vi "MEASURE_2dmapping-2.vi"() -> ()   [LabVIEW 2021]
uses:
  <vilib>/Math Plots/3D Math Plots/3D Surface/3D Surface XCtrl/3D Surface.xctl
  <vilib>/Math Plots/3D Math Plots/3D Surface/3D Surface Datatype/3D Surface Datatype.lvclass
  <instrlib>/Keithley 24XX/Public/Data/Read (Multiple Points).vi
  <vilib>/Utility/file.llb/Write To Spreadsheet File (DBL).vi
  <vilib>/Math Plots/3D Math Plots/3D Surface/3D Surface Datatype/Public/Plot Helper (Vector).vi
  <instrlib>/Stanford Research 830/Stanford Research 830.lvlib
  <instrlib>/Keithley 2450/Keithley 2450.lvlib
  <instrlib>/Keithley 24XX/Keithley 24XX.lvlib
  <vilib>/Analysis/NI_AALBase.lvlib
panel:
  in  "manual phase 2":dbl=1.0
  in  "auto phase 2":bool=TRUE
  in  "harmonic 2":dbl=1.0
  in  "Sine Output Amplitude (1 V) 3":dbl=0.05
  in  "Input Connection (0: Single-Ended Voltage)  2":u16(ring) items=["Single-Ended Voltage", "Differential Voltage", "1 MOhm Current Gain", "100 MOhm Current Gain"]
  in  "frequency 2":dbl=50.0 format="%#_13g"
  in  "manual phase":dbl=1.0
  in  "auto phase":bool=TRUE
  in  "harmonic":dbl=1.0
  in  "LOCKIN address 2":refnum<visa-resource-name>="GPIB0::8::INSTR"
  in  "GATE / SD stablization 5":dbl=0.1 format="%#_13g"
  in  "GATE / SD stablization 4":dbl=0.1 format="%#_13g"
  in  "ramping step":i32=20
  in  "Compliance  Level (1uA) 2":dbl=1e-08
  in  "Source Mode  (0: Voltage) 2":u16(ring) items=["Voltage", "Current"]
  out "3D Surface":refnum<class "3D Plot Datatype.lvclass">[](xcontrol)
  in  "scaning step2":i32=60
  out "gate voltage1":dbl=3.0 format="%#_13g"
  in  "scanning step1":i32=30
  in  "GATE2 end Value   2":dbl=10.0
  in  "GATE2 starting Value  2":dbl=-14.0
  out "gate 2leaking":dbl=1.1399661770106206e-10
  out "gate voltage2":dbl=10.0 format="%#_13g"
  in  "Serial Configuration":T1={"Baud Rate"=9600, "Parity"=0, "Data Bits"=8, "Stop Bits"=10, "Flow Control"=0} {"Flow Control" items=["None", "XON/XOFF", "RTS/CTS", "XON/XOFF & RTS/CTS", "DTR/DSR", "XON/XOFF & DTR/DSR"]; "Stop Bits" items=["1.0"=10, "1.5"=15, "2.0"=20]; "Data Bits" items=["7"=7, "8"=8]; "Parity" items=["None", "Odd", "Even", "Mark", "Space"]; "Baud Rate" items=["300"=300, "600"=600, "1200"=1200, "2400"=2400, "4800"=4800, "9600"=9600, "19200"=19200]}
  in  "gate2 address":refnum<visa-resource-name>="GPIB0::25::INSTR"
  in  "Save data or not":bool=TRUE
  in  "path (folder + filename)":string="C:\\Users\\User\\Data\\Jason\\03282019\\mapping_3"
  out "XY Graph":cluster{dbl[], dbl[]}(graph)={[-14.0, -13.6, -13.2, -12.8, -12.4, -12.0, -11.6, -11.2, -10.8, -10.4, -10.0, -9.6, -9.2, -8.8, -8.399999999999999, -8.0, -7.6, -7.199999999999999, -6.8, -6.3999999999999995, -6.0, -5.6, -5.199999999999999, -4.799999999999999, -4.399999999999999, -4.0, -3.5999999999999996, -3.1999999999999993, -2.799999999999999, -2.3999999999999986, -2.0, -1.5999999999999996, -1.1999999999999993, -0.7999999999999989, -0.3999999999999986, 0.0, 0.40000000000000036, 0.8000000000000007, 1.200000000000001, 1.6000000000000014, 2.0, 2.400000000000002, 2.8000000000000007, 3.1999999999999993, 3.6000000000000014, 4.0, 4.400000000000002, 4.800000000000001, 5.200000000000003, 5.600000000000001, 6.0, 6.400000000000002, 6.800000000000001, 7.200000000000003, 7.600000000000001, 8.0, 8.400000000000002, 8.8, 9.200000000000003, 9.600000000000001, 10.0], [0.000948314, 0.000947837, 0.000947598, 0.000947479, 0.000947241, 0.000946883, 0.000946645, 0.000945572, 0.000944141, 0.000942711, 0.000941519, 0.000939969, 0.000938658, 0.000937108, 0.00093532, 0.000933651, 0.000931863, 0.000929955, 0.000928048, 0.000926021, 0.000923995, 0.00092173, 0.000919465, 0.0009172, 0.000914697, 0.000912312, 0.000909809, 0.000907306, 0.000904683, 0.00090218, 0.000899557, 0.000896934, 0.000894193, 0.00089157, 0.000888947, 0.000886325, 0.000883702, 0.00088108, 0.000878457, 0.000875834, 0.000873331, 0.000870828, 0.000868324, 0.00086594, 0.000863437, 0.000861172, 0.000858787, 0.000856522, 0.000854257, 0.000852112, 0.000849966, 0.000847939, 0.000846032, 0.000844125, 0.000842217, 0.000840429, 0.000838879, 0.000837211, 0.000835661, 0.00083435, 0.000833277]}
  out "LOCKIN Measurement":dbl=0.000833277
  in  "Parameter (1: X)":u16(ring)=1 items=["X"=1, "Y"=2, "R"=3, "Theta"=4, "Channel 1"=5, "Channel 2"=6, "Aux In 1"=7, "Aux In 2"=8, "Aux In 3"=9, "Aux In 4"=10]
  out "gate leaking":string="4.458176E-12\n"
  in  "GATE1 end Value (default 0)":dbl=3.0
  in  "GATE1 starting(small) Value":dbl=-3.0
  in  "Function (0: Volts) 2":u16(ring) items=["Volts", "Current", "Resistance"]
  in  "Source Compaliance":dbl=1e-08
  in  "gate1 address":refnum<visa-resource-name>="GPIB0::18::INSTR"
  in  "SD stabilization(S) 2":dbl=0.1 format="%#_13g"
  in  "Sine Output Amplitude (1 V) 2":dbl=0.05
  in  "GATE / SD stablization 3":dbl=0.2 format="%#_13g"
  in  "frequency":dbl=50.0 format="%#_13g"
  in  "Input Connection (0: Single-Ended Voltage)":u16(ring) items=["Single-Ended Voltage", "Differential Voltage", "1 MOhm Current Gain", "100 MOhm Current Gain"]
  in  "LOCKIN address":refnum<visa-resource-name>="GPIB0::8::INSTR"
  # "Lock-in"
  # "2450 Gate Setting"
  # "2401 Gate Setting"
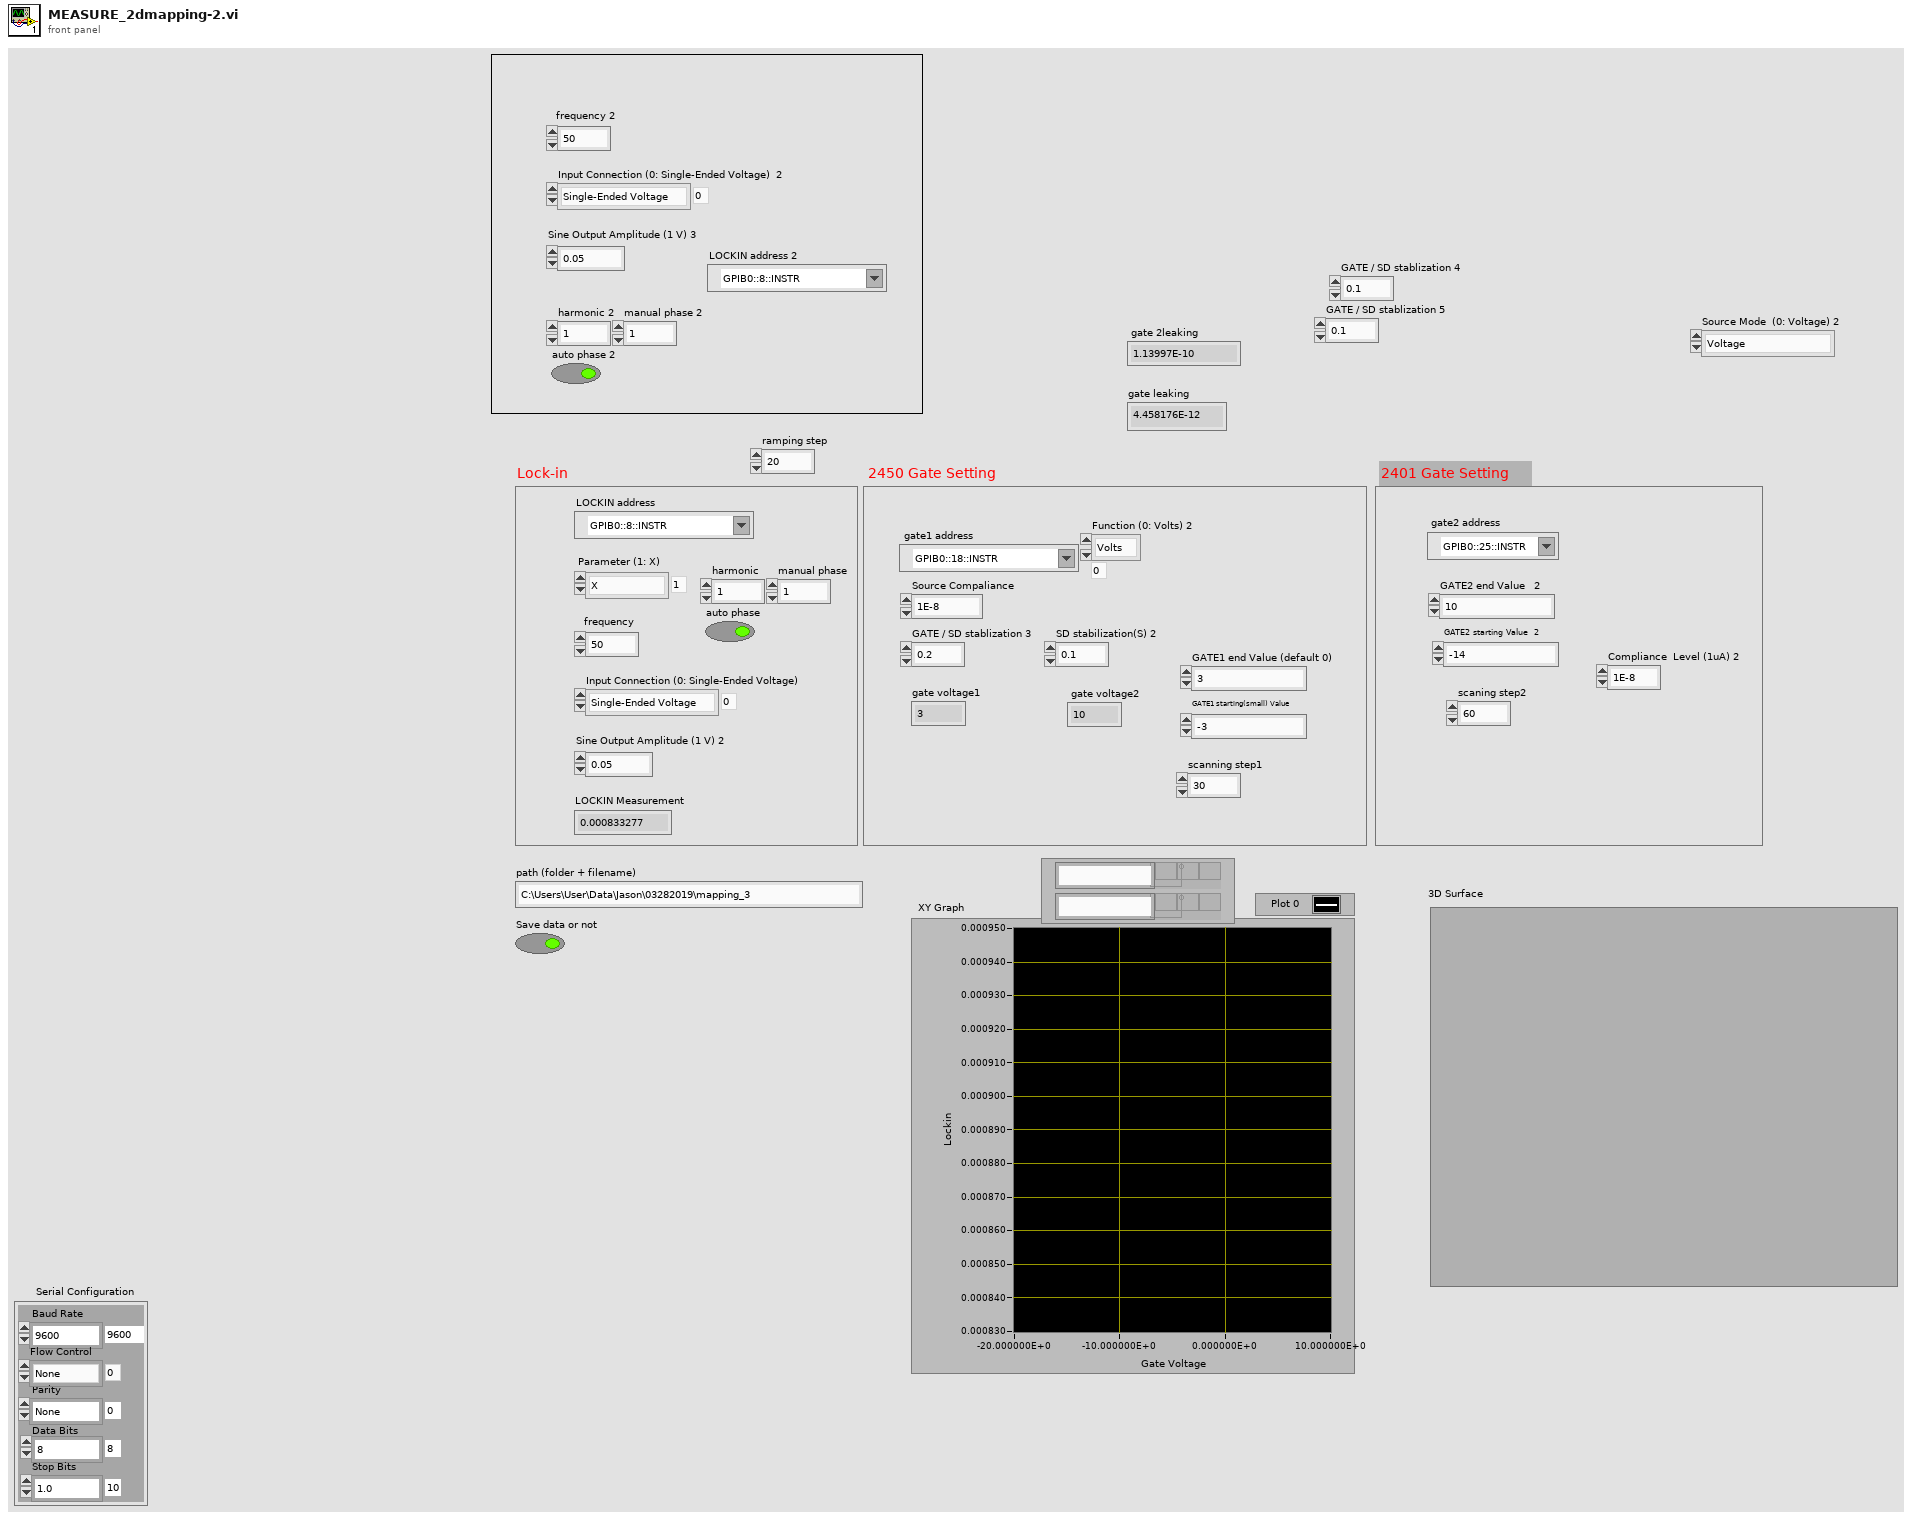
[diagram p1: front panel]
types:
  T1 = cluster{"Baud Rate":u32, "Parity":u16, "Data Bits":u16, "Stop Bits":u16, "Flow Control":u16}
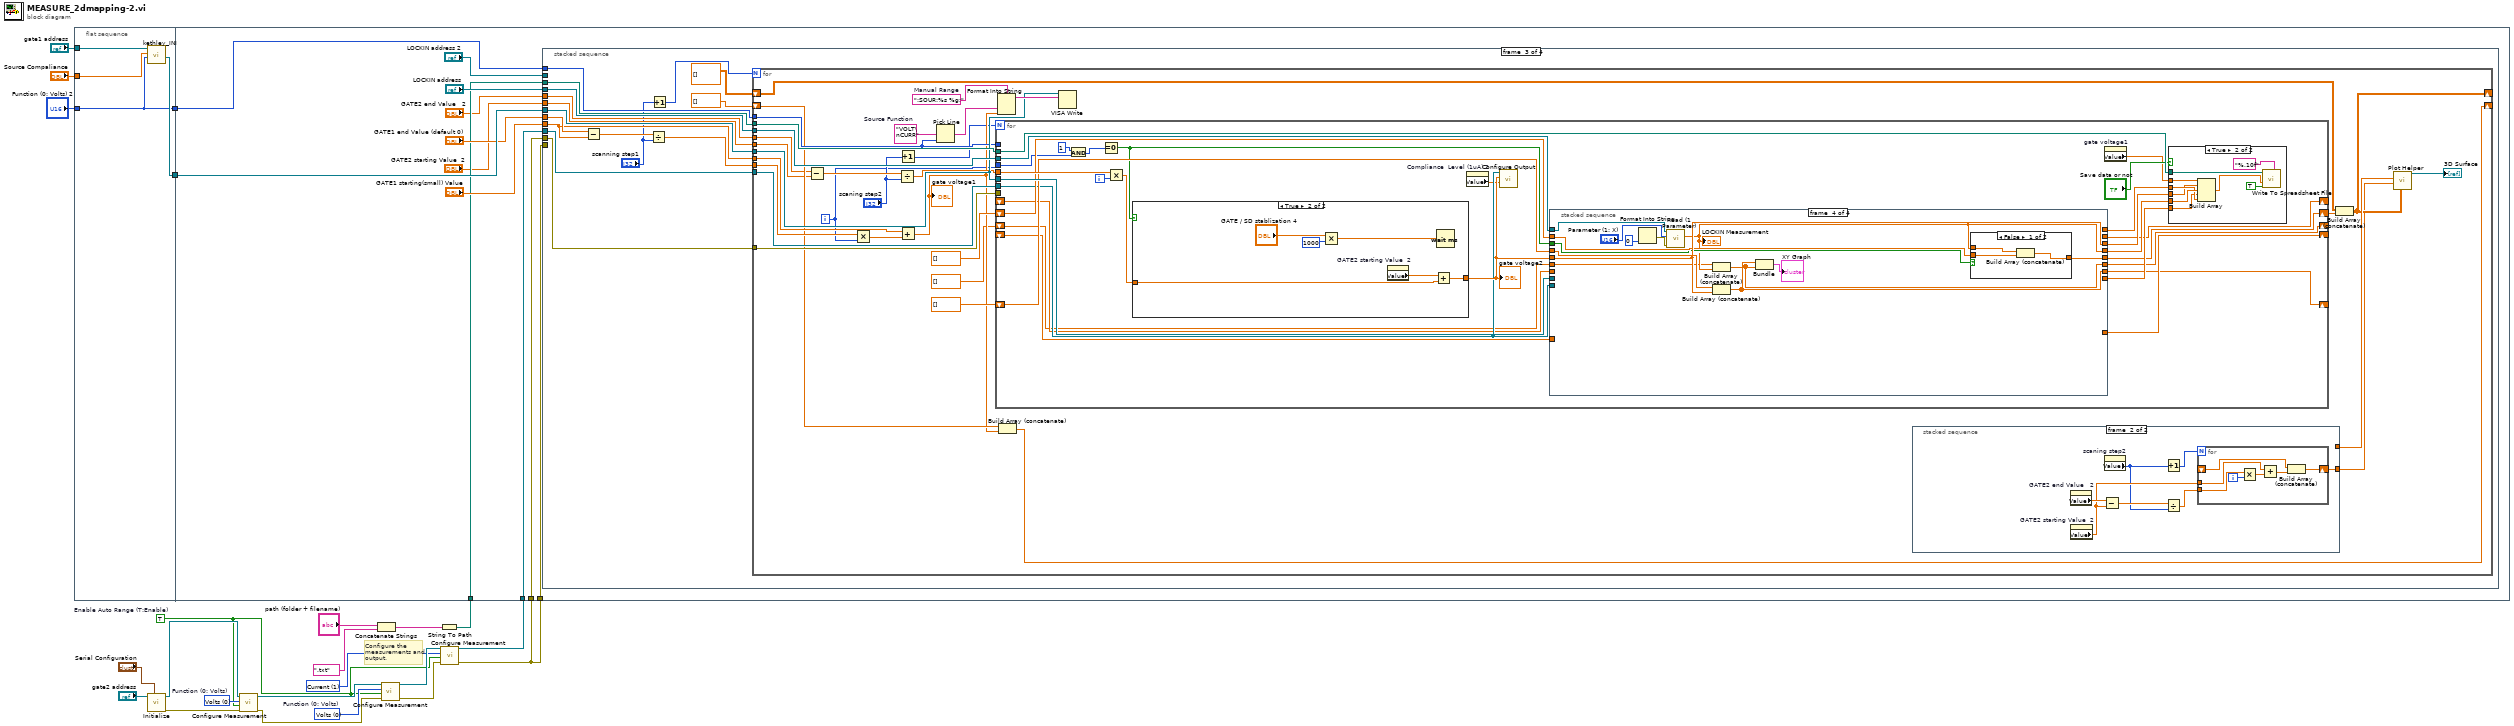
[diagram p0: block diagram]
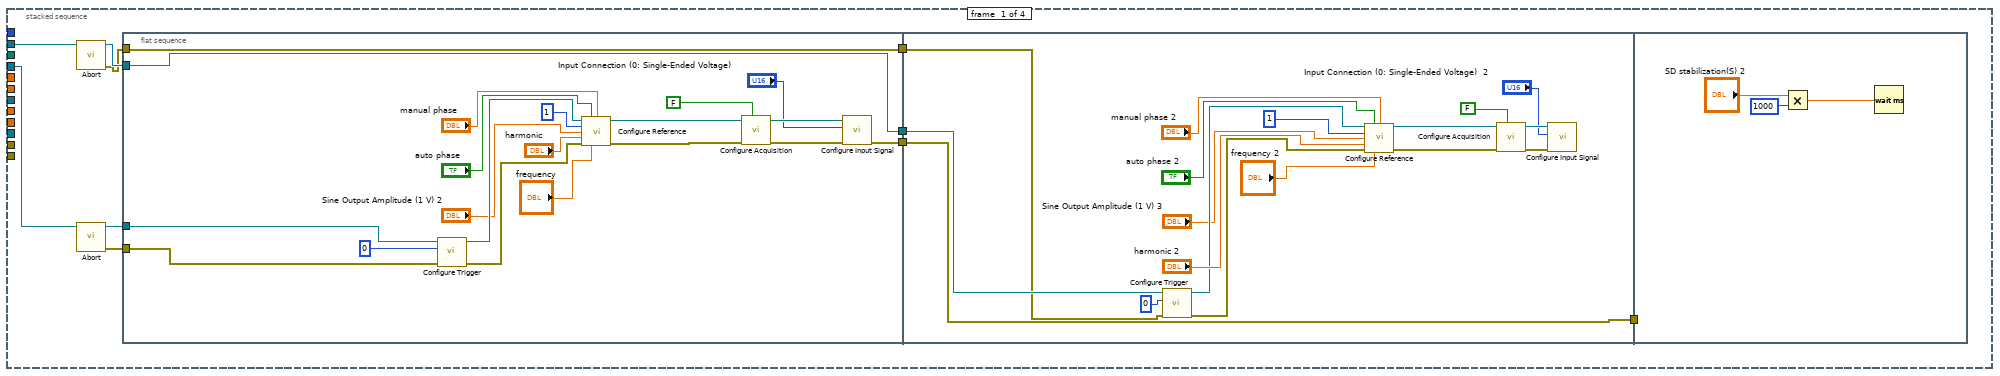
[diagram p2: hidden frame]
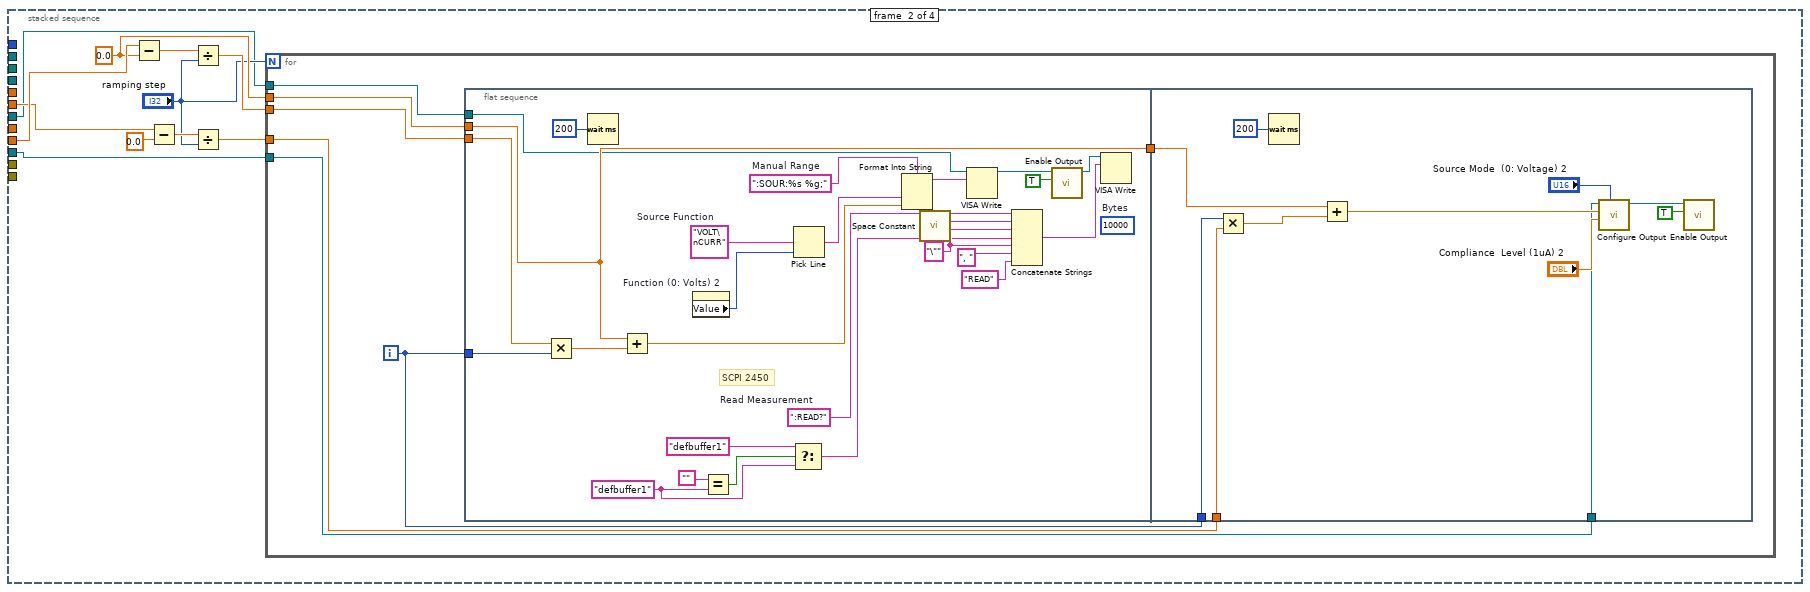
[diagram p3: hidden frame]
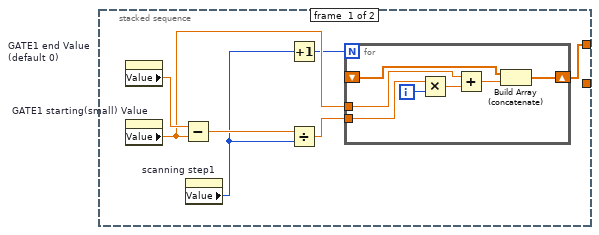
[diagram p4: hidden frame]
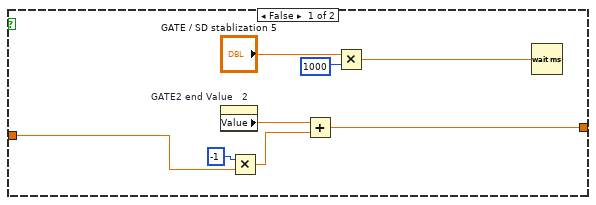
[diagram p5: hidden frame]
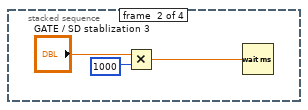
[diagram p8: hidden frame]
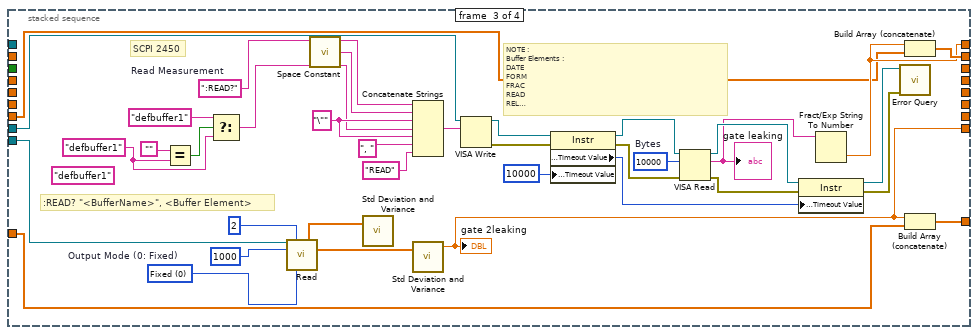
[diagram p9: hidden frame]
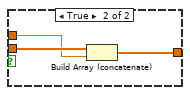
[diagram p10: hidden frame]
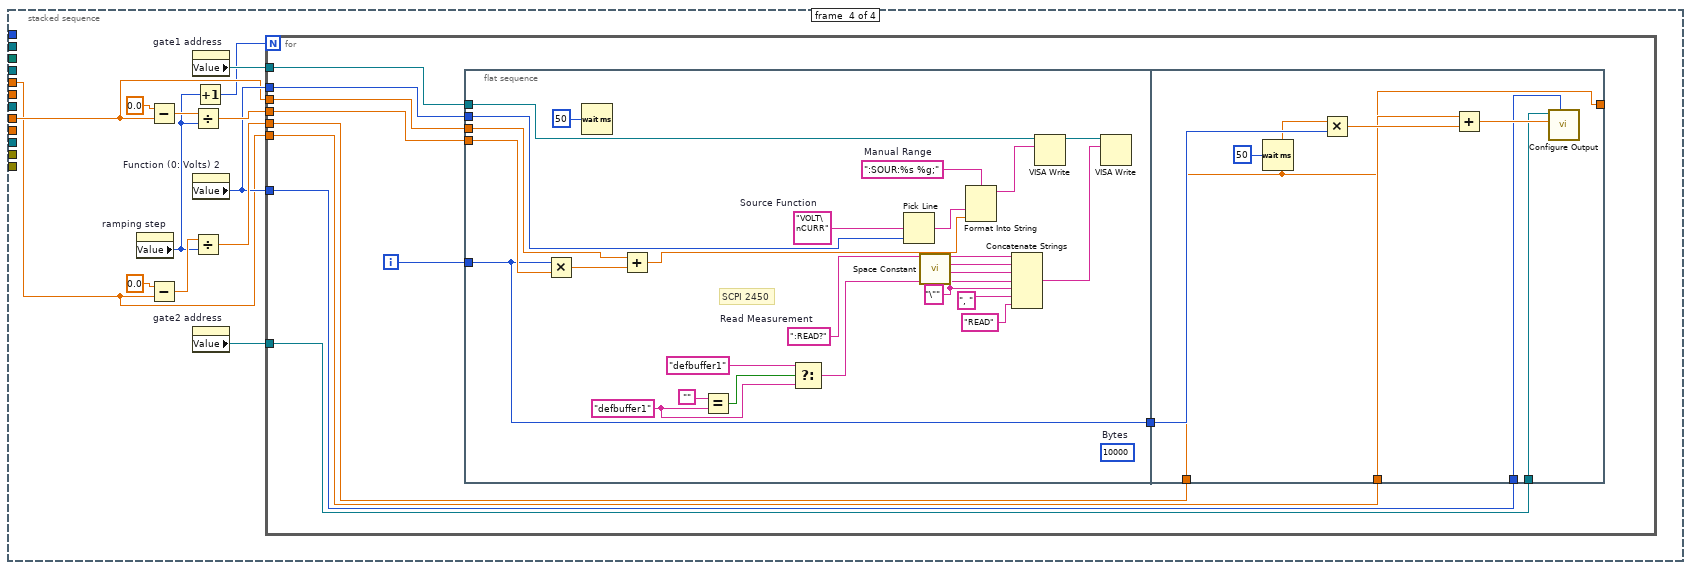
[diagram p11: hidden frame]
diagram:
  w3 = u16 1 items=["Volts", "Current", "Resistance"] ("Function (0: Volts)")
  w4 = TRUE  # Enable Auto Range (T:Enable)
  w7 = u16 0 items=["Volts", "Current", "Resistance"]  # Function (0: Volts)
  w8 = u16 0 items=["Volts", "Current", "Resistance"]  # Function (0: Volts)
  # "Configure the measurements and output."
  n1 = flat-sequence {
    tunnel: "gate1 address" -> [w27]
    tunnel: "Source Compaliance" -> [w26]
    tunnel: "Function (0: Volts) 2" -> [w24]
    tunnel: [w25] -> w20
    tunnel: [w24] -> w19
    tunnel: w20 -> [w38]
    tunnel: w19 -> [w37]
    tunnel: w15 -> [w34]
    tunnel: w2 -> [w33]
    tunnel: w1 -> [w32]
    tunnel: w1 -> [w29]
    frame #0 {
      n2 = call "kethley_INI.vi"("Function (0: Volts) in"=w24, "Source Compaliance"=w26, "VISA Refnum in"=w27) -> ("VISA resource name out"=w25:refnum<visa-resource-name>)  [unwired: 8 in]
    }
    frame #1 {
      n3 = stacked-sequence {
        tunnel: "LOCKIN address" -> [w49 _ w161 _]
        tunnel: w38 -> [_ w92 w158 _]
        tunnel: w37 -> [_ _ w157 _]
        tunnel: "GATE1 starting(small) Value" -> [_ w99 w151 _]
        tunnel: "GATE1 end Value (default 0)" -> [_ _ w152 w337]
        tunnel: w34 -> [_ _ w160 _]
        tunnel: w33 -> [_ w91 w156 _]
        tunnel: w32 -> [_ _ w159 _]
        tunnel: "GATE2 starting Value  2" -> [_ w94 w149 _]
        tunnel: "GATE2 end Value   2" -> [_ _ w150 w335]
        tunnel: w29 -> [_ _ _ _]
        tunnel: "LOCKIN address 2" -> [w43 _ _ _]
        frame #0 {
          n4 = call <instrlib>:"Abort.vi"("VISA resource name"=w43) -> ("error out"=w40:errorcluster, "VISA resource name out"=w42:refnum<visa-resource-name>)  [unwired: 9 in]
          n5 = call <instrlib>:"Abort.vi"("VISA resource name"=w49) -> ("error out"=w47:errorcluster, "VISA resource name out"=w48:refnum<visa-resource-name>)  [unwired: 9 in]
          n6 = flat-sequence {
            tunnel: w48 -> [w69]
            tunnel: [w54] -> w46
            tunnel: w47 -> [w53]
            tunnel: w42 -> [w51]
            tunnel: [w51] -> w44
            tunnel: [w50] -> w41
            tunnel: w40 -> [w50]
            tunnel: w46 -> [w87]
            tunnel: [w87] -> w45
            tunnel: w44 -> [w71]
            tunnel: w41 -> [w70]
            tunnel: w45 -> [_]
            frame #0 {
              n7 = call <instrlib>:"Configure Trigger.vi"("error in (no error)"=w53, "Trigger Source (0: Internal)"=0, "VISA resource name"=w69) -> ("error out"=w63:errorcluster, "VISA resource name out"=w64:refnum<visa-resource-name>)  [unwired: 7 in]
              n8 = call <instrlib>:"Configure Reference.vi"("VISA resource name"=w64, "Auto Phase (T: Enabled)"="auto phase", "Manual Phase (0 Degree)"="manual phase", "Reference Source (1: Internal)"=1, "Sine Output Amplitude (1 V)"="Sine Output Amplitude (1 V) 2", "Detection Harmonic Number (1)"="harmonic", "error in (no error)"=w63, "Internal Reference Frequency (1000 Hz)"="frequency") -> ("VISA resource name out"=w61:refnum<visa-resource-name>, "error out"=w56:errorcluster)  [unwired: 6 in]
              n9 = call <instrlib>:"Configure Acquisition.vi"("Continuous Storage (T: Enable)"=FALSE, "error in (no error)"=w56, "VISA resource name"=w61) -> ("error out"=w55:errorcluster, "VISA resource name out"=w59:refnum<visa-resource-name>)  [unwired: 7 in]
              n10 = call <instrlib>:"Configure Input Signal.vi"("error in (no error)"=w55, "Input Connection (0: Single-Ended Voltage)"="Input Connection (0: Single-Ended Voltage)", "VISA resource name"=w59) -> ("error out"=w54:errorcluster)  [unwired: 7 in, 1 out]
            }
            frame #1 {
              n11 = call <instrlib>:"Configure Trigger.vi"("error in (no error)"=w70, "Trigger Source (0: Internal)"=0, "VISA resource name"=w71) -> ("error out"=w81:errorcluster, "VISA resource name out"=w82:refnum<visa-resource-name>)  [unwired: 7 in]
              n12 = call <instrlib>:"Configure Reference.vi"("VISA resource name"=w82, "Auto Phase (T: Enabled)"="auto phase 2", "Manual Phase (0 Degree)"="manual phase 2", "Reference Source (1: Internal)"=1, "Sine Output Amplitude (1 V)"="Sine Output Amplitude (1 V) 3", "Detection Harmonic Number (1)"="harmonic 2", "error in (no error)"=w81, "Internal Reference Frequency (1000 Hz)"="frequency 2") -> ("VISA resource name out"=w79:refnum<visa-resource-name>, "error out"=w74:errorcluster)  [unwired: 6 in]
              n13 = call <instrlib>:"Configure Acquisition.vi"("Continuous Storage (T: Enable)"=FALSE, "error in (no error)"=w74, "VISA resource name"=w79) -> ("error out"=w73:errorcluster, "VISA resource name out"=w77:refnum<visa-resource-name>)  [unwired: 7 in]
              n14 = call <instrlib>:"Configure Input Signal.vi"("error in (no error)"=w73, "Input Connection (0: Single-Ended Voltage)"="Input Connection (0: Single-Ended Voltage)  2", "VISA resource name"=w77) -> ()  [unwired: 7 in, 2 out]
            }
            frame #2 {
              n15 = Multiply(x="SD stabilization(S) 2", y=1000) -> (x*y=w90:dbl)
              n16 = Wait (ms)(milliseconds to wait=w90) -> ()  [unwired: 1 out]
            }
          }
        }
        frame #1 {
          w98 = 0.0
          n17 = Subtract(x=w99, y=w98) -> (x-y=w101:dbl)
          n18 = Subtract(x=w94, y=0.0) -> (x-y=w97:dbl)
          n19 = Divide(x=w101, y="ramping step") -> (x/y=w100:dbl)
          n20 = Divide(x=w97, y="ramping step") -> (x/y=w93:dbl)
          n21 = for {
            N: "ramping step" -> [_]
            tunnel: w100 -> [w108]
            tunnel: w98 -> [w107]
            tunnel: w93 -> [w106]
            tunnel: w92 -> [w103]
            tunnel: w91 -> [w102]
            i -> [w105]
            n22 = flat-sequence {
              tunnel: w105 -> [w128]
              tunnel: w108 -> [w127]
              tunnel: w107 -> [w126]
              tunnel: [w126] -> w104
              tunnel: w103 -> [w124]
              tunnel: w106 -> [w142]
              tunnel: w105 -> [w141]
              tunnel: w104 -> [w140]
              tunnel: w102 -> [w138]
              frame #0 {
                w109 = "defbuffer1" ("Buffer Name (defbuffer1) 2")
                w117 = "\""
                w114 = ":READ?"  # Read Measurement
                (unwired) u32 10000  # Bytes
                w133 = "VOLT\nCURR"  # Source Function
                w132 = ":SOUR:%s %g;"  # Manual Range
                # "SCPI 2450"
                n23 = Multiply(x=w127, y=w128) -> (x*y=w130:dbl)
                n24 = Wait (ms)(milliseconds to wait=200) -> ()  [unwired: 1 out]
                n25 = Add(x=w126, y=w130) -> (x+y=w129:dbl)
                n26 = property on="Function (0: Volts) 2" class="Ring (strict)"() -> ("Value"=w125:u16)  [unwired: 2 in, 2 out]
                n27 = Equal?(x="", y=w109) -> (x = y?=w110:bool)
                n28 = Select(t="defbuffer1", s=w110, f=w109) -> (s? t:f=w116:string)
                n29 = Pick Line(multi-line string=w133, line index=w125) -> (output string=w134:string)  [unwired: 1 out]
                n30 = Format Into String(format string=w132, w134, w129) -> (resulting string=w131:string)  [unwired: 2 in, 1 out]
                n31 = call <vilib>:"Space Constant.vi"() -> ("String"=w115:string)
                n32 = VISA Write(VISA resource name=w124, write buffer=w131) -> (VISA resource name out=w122:refnum<visa-resource-name>)  [unwired: 1 in, 2 out]
                n33 = Concatenate Strings(w114, w115, w117, w116, w117, ", " ("string"), "READ" ("Buffer Elements 2")) -> (w120:string)
                n34 = call <instrlib>:"Enable Output.vi"("Enable Output (T: Enable)"=TRUE, "VISA resource name"=w122) -> ("VISA resource name out"=w111:refnum<visa-resource-name>)  [unwired: 8 in, 1 out]
                n35 = VISA Write(VISA resource name=w111, write buffer=w120) -> ()  [unwired: 1 in, 3 out]
              }
              frame #1 {
                n36 = Multiply(x=w141, y=w142) -> (x*y=w143:dbl)
                n37 = Wait (ms)(milliseconds to wait=200) -> ()  [unwired: 1 out]
                n38 = Add(x=w140, y=w143) -> (x+y=w144:dbl)
                n39 = call <instrlib>:"Configure Output.vi"("Source Mode  (0: Voltage)"="Source Mode  (0: Voltage) 2", "Compliance  Level (0.1)"="Compliance  Level (1uA) 2", "Output Level (0)"=w144, "VISA resource name"=w138) -> ("VISA resource name out"=w135:refnum<visa-resource-name>)  [unwired: 6 in, 1 out]
                n40 = call <instrlib>:"Enable Output.vi"("Enable Output (T: Enable)"=TRUE, "VISA resource name"=w135) -> ()  [unwired: 8 in, 2 out]
              }
            }
          }
        }
        frame #2 {
          n41 = Subtract(x=w152, y=w151) -> (x-y=w155:dbl)
          n42 = Divide(x=w155, y="scanning step1") -> (x/y=w154:dbl)
          n43 = Increment(x="scanning step1") -> (x+1=w147:i32)
          n44 = for {
            N: w147 -> [_]
            tunnel: w157 -> [w181]
            tunnel: w158 -> [w182]
            tunnel: w161 -> [w193]
            tunnel: w160 -> [w192]
            tunnel: w159 -> [w191]
            tunnel: w156 -> [w190]
            tunnel: w151 -> [w189]
            tunnel: w154 -> [w188]
            shift-right: [w164] -> _
            shift-left: dbl[] [] ("appended array") -> [w176]
            tunnel: w150 -> [w173]
            tunnel: w149 -> [w172]
            shift-right: [w165] -> _
            shift-left: dbl[][] [] ("Intensity Graph") -> [w166]
            i -> [w169]
            w184 = "VOLT\nCURR"  # Source Function
            w185 = ":SOUR:%s %g;"  # Manual Range
            n45 = Subtract(x=w173, y=w172) -> (x-y=w180:dbl)
            n46 = Multiply(x=w188, y=w169) -> (x*y=w187:dbl)
            n47 = Divide(x=w180, y="scaning step2") -> (x/y=w179:dbl)
            n48 = Increment(x="scaning step2") -> (x+1=w170:i32)
            n49 = Add(x=w189, y=w187) -> (x+y=w175:dbl)
            "gate voltage1" <- w175
            n50 = Pick Line(multi-line string=w184, line index=w181) -> (output string=w183:string)  [unwired: 1 out]
            n51 = for {
              N: w170 -> [_]
              tunnel: w181 -> [_]
              tunnel: w182 -> [w250]
              tunnel: w193 -> [w249]
              tunnel: w192 -> [w246]
              tunnel: w191 -> [_]
              tunnel: w190 -> [w234]
              shift-right: [w237] -> _
              shift-left: _ -> [w224]
              tunnel: w179 -> [w243]
              shift-right: [w239] -> w174
              shift-left: dbl[] [] ("appended array") -> [w240]
              shift-right: [w227] -> _
              shift-left: dbl[] [] ("appended array") -> [w238]
              shift-right: [w233] -> _
              shift-left: _ -> [w232]
              tunnel: w169 -> [w228]
              shift-right: [w225] -> _
              shift-left: dbl[] [] ("appended array") -> [w223]
              i -> [w230]
              n52 = And(x=1, y=w228) -> (x .and. y?=w229:i32)
              n53 = Equal To 0?(x=w229) -> (x = 0?=w226:bool)
              n54 = Multiply(x=w243, y=w230) -> (x*y=w242:dbl)
              n55 = case shown="True" w226 {
                tunnel: w242 -> [w258 w259]
                tunnel: [w254 w263] -> w241
                frame False {
                  n56 = property on="GATE2 end Value   2" class="DigNum (strict)"() -> ("Value"=w255:dbl)  [unwired: 2 in, 2 out]
                  n57 = Multiply(x=-1, y=w258) -> (x*y=w256:dbl)
                  n58 = Add(x=w255, y=w256) -> (x+y=w254:dbl)
                  n59 = Multiply(x="GATE / SD stablization 5", y=1000) -> (x*y=w253:dbl)
                  n60 = Wait (ms)(milliseconds to wait=w253) -> ()  [unwired: 1 out]
                }
                frame True {
                  n61 = Multiply(x="GATE / SD stablization 4", y=1000) -> (x*y=w262:dbl)
                  n62 = property on="GATE2 starting Value  2" class="DigNum (strict)"() -> ("Value"=w264:dbl)  [unwired: 2 in, 2 out]
                  n63 = Add(x=w264, y=w259) -> (x+y=w263:dbl)
                  n64 = Wait (ms)(milliseconds to wait=w262) -> ()  [unwired: 1 out]
                }
              }
              "gate voltage2" <- w241
              n65 = property on="Compliance  Level (1uA) 2" class="DigNum (strict)"() -> ("Value"=w222:dbl)  [unwired: 2 in, 2 out]
              n66 = call <instrlib>:"Configure Output.vi"("Compliance  Level (0.1)"=w222, "Output Level (0)"=w241, "VISA resource name"=w234) -> ()  [unwired: 7 in, 2 out]
              n67 = stacked-sequence {
                tunnel: w250 -> [_ _ w290 _]
                tunnel: w249 -> [_ _ _ w323]
                tunnel: [_ _ w289 _] -> w233
                tunnel: w240 -> [_ _ _ w318]
                tunnel: [_ _ _ w317] -> w239
                tunnel: [_ _ _ w321] -> w227
                tunnel: [_ _ _ w315] -> w248
                tunnel: [_ _ w287 _] -> w247
                tunnel: [_ _ w281 _] -> w237
                tunnel: w224 -> [_ _ w280 _]
                tunnel: [_ _ w279 _] -> w244
                tunnel: w241 -> [_ _ _ w319]
                tunnel: w238 -> [_ _ _ w320]
                tunnel: [_ _ _ w319] -> w236
                tunnel: w234 -> [_ _ w277 _]
                tunnel: w232 -> [_ _ w278 _]
                tunnel: w226 -> [_ _ _ w316]
                tunnel: [_ _ _ w313] -> w225
                tunnel: w223 -> [_ _ _ w314]
                frame #0 {
                }
                frame #1 {
                  n68 = Multiply(x="GATE / SD stablization 3", y=1000) -> (x*y=w276:dbl)
                  n69 = Wait (ms)(milliseconds to wait=w276) -> ()  [unwired: 1 out]
                }
                frame #2 {
                  w284 = u16 0 items=["Fixed", "Sweep", "List"]  # Output Mode (0: Fixed)
                  w301 = "defbuffer1" ("Buffer Name (defbuffer1) 2")
                  (unwired) "defbuffer1" ("t")
                  w299 = "\""
                  w296 = ":READ?"  # Read Measurement
                  w305 = u32 10000  # Bytes
                  # "NOTE :\nBuffer Elements :\nDATE\nFORM\nFRAC\nREAD\nREL\nSEC\nSOUR\nSOURFORM\nSOURSTAT\nSOURUNIT\nSTAT\nTIME\nTsT\nUNIT"
                  # ":READ? \"<BufferName>\", <Buffer Element>"
                  # "SCPI 2450"
                  n70 = Equal?(x="", y=w301) -> (x = y?=w302:bool)
                  n71 = Select(t="defbuffer1", s=w302, f=w301) -> (s? t:f=w298:string)
                  n72 = call-poly <instrlib>:"Read.vi"("VISA resource name"=w277, "Sample Count (1)"=u32 2 ("Number of Samples"), "Timeout (10000 ms)"=1000, "Output Mode (0: Fixed)"=w284) -> ("Voltage"=w282:sgl[], "Current"=w283:sgl[])  [unwired: 5 in, 5 out]
                  n73 = call <vilib>:"Space Constant.vi"() -> ("String"=w297:string)
                  n74 = call <vilib>:"Std Deviation and Variance.vi"("X"=w282) -> ()  [unwired: 1 in, 3 out]
                  n75 = Concatenate Strings(w296, w297, w299, w298, w299, ", " ("string"), "READ" ("Buffer Elements 2")) -> (w312:string)
                  n76 = call <vilib>:"Std Deviation and Variance.vi"("X"=w283) -> ("mean"=w279:dbl)  [unwired: 1 in, 2 out]
                  "gate 2leaking" <- w279
                  n77 = VISA Write(VISA resource name=w290, write buffer=w312) -> (VISA resource name out=w304:refnum<visa-resource-name>, error out=w311:errorcluster)  [unwired: 1 in, 1 out]
                  n78 = property class="Instr"(reference=w304, error in=w311, "General Settings:Timeout Value"=10000 ("Timeout (10000 ms) 2")) -> (reference out=w310:refnum<visa-resource-name>, error out=w309:errorcluster, "General Settings:Timeout Value"=w306:u32)
                  n79 = VISA Read(VISA resource name=w310, byte count=w305, error in (no error)=w309) -> (VISA resource name out=w308:refnum<visa-resource-name>, read buffer=w288:string, error out=w307:errorcluster)  [unwired: 1 out]
                  "gate leaking" <- w288
                  n80 = property class="Instr"(reference=w308, error in=w307, "General Settings:Timeout Value"=w306) -> (reference out=w294:refnum<visa-resource-name>, error out=w293:errorcluster)
                  n81 = Fract/Exp String To Number(string=w288) -> (number=w287:dbl)  [unwired: 3 in, 1 out]
                  n82 = call <instrlib>:"Error Query.vi"("error in (no error)"=w293, "VISA resource name"=w294) -> ()  [unwired: 10 out]
                  n83 = Build Array (concatenate)(w287, w278) -> (w289:dbl[])
                  n84 = Build Array (concatenate)(w279, w280) -> (w281:dbl[])
                }
                frame #3 {
                  n85 = Format Into String(0) -> (error out=w326:errorcluster)  [unwired: 3 in, 1 out]
                  n86 = call <instrlib>:"Read (1 Parameter).vi"("error in (no error)"=w326, "Parameter (1: X)"="Parameter (1: X)", "VISA resource name"=w323) -> ("Measurement"=w315:dbl)  [unwired: 6 in, 2 out]
                  "LOCKIN Measurement" <- w315
                  n87 = Build Array (concatenate)(w314, w315) -> (w313:dbl[])
                  n88 = Build Array (concatenate)(w320, w319) -> (w321:dbl[])
                  n89 = Bundle(w321, w313) -> (→"XY Graph":cluster{dbl[], dbl[]})  [unwired: 1 in]
                  n90 = case shown="False" w316 {
                    tunnel: w318 -> [w328 w332]
                    tunnel: w315 -> [w329 w331]
                    tunnel: [w327 w330] -> w317
                    frame False {
                      n91 = Build Array (concatenate)(w329, w328) -> (w327:dbl[])
                    }
                    frame True {
                      n92 = Build Array (concatenate)(w332, w331) -> (w330:dbl[])
                    }
                  }
                }
              }
              n93 = property on="gate voltage1" class="DigNum (strict)"() -> ("Value"=w235:dbl)  [unwired: 2 in, 2 out]
              n94 = case shown="True" "Save data or not" {
                tunnel: w248 -> [_ w273]
                tunnel: w247 -> [_ w272]
                tunnel: w246 -> [_ w270]
                tunnel: w244 -> [_ w267]
                tunnel: w236 -> [_ w266]
                tunnel: w235 -> [_ w265]
                frame False {
                }
                frame True {
                  n95 = Build Array(w265, w266, w273, w267, w272) -> (w271:dbl[])
                  n96 = call-poly <vilib>:"Write To Spreadsheet File.vi"("format (%.3f)"="%.10f", "append to file? (new file:F)"=TRUE, "1D data"=w271, "file path (dialog if empty)"=w270) -> ()  [unwired: 4 in, 1 out]
                }
              }
            }
            n97 = Format Into String(format string=w185, w183, w175) -> (resulting string=w186:string)  [unwired: 2 in, 1 out]
            n98 = Build Array (concatenate)(w176, w175) -> (w164:dbl[])
            n99 = VISA Write(VISA resource name=w182, write buffer=w186) -> ()  [unwired: 1 in, 3 out]
            n100 = stacked-sequence {
              tunnel: [w196 _] -> w167
              tunnel: [_ w210] -> w162
              frame #0 {
                n101 = property on="GATE1 end Value (default 0)" class="DigNum (strict)"() -> ("Value"=w200:dbl)  [unwired: 2 in, 2 out]
                n102 = property on="GATE1 starting(small) Value" class="DigNum (strict)"() -> ("Value"=w197:dbl)  [unwired: 2 in, 2 out]
                n103 = Subtract(x=w200, y=w197) -> (x-y=w199:dbl)
                n104 = property on="scanning step1" class="DigNum (strict)"() -> ("Value"=w195:i32)  [unwired: 2 in, 2 out]
                n105 = Increment(x=w195) -> (x+1=w194:i32)
                n106 = Divide(x=w199, y=w195) -> (x/y=w198:dbl)
                n107 = for {
                  N: w194 -> [_]
                  tunnel: w198 -> [w206]
                  tunnel: w197 -> [w204]
                  shift-right: [w203] -> w196
                  shift-left: _ -> [w202]
                  i -> [w207]
                  n108 = Multiply(x=w206, y=w207) -> (x*y=w205:dbl)
                  n109 = Add(x=w204, y=w205) -> (x+y=w201:dbl)
                  n110 = Build Array (concatenate)(w202, w201) -> (w203:dbl[])
                }
              }
              frame #1 {
                n111 = property on="GATE2 end Value   2" class="DigNum (strict)"() -> ("Value"=w213:dbl)  [unwired: 2 in, 2 out]
                n112 = property on="GATE2 starting Value  2" class="DigNum (strict)"() -> ("Value"=w212:dbl)  [unwired: 2 in, 2 out]
                n113 = Subtract(x=w213, y=w212) -> (x-y=w211:dbl)
                n114 = property on="scaning step2" class="DigNum (strict)"() -> ("Value"=w209:i32)  [unwired: 2 in, 2 out]
                n115 = Increment(x=w209) -> (x+1=w208:i32)
                n116 = Divide(x=w211, y=w209) -> (x/y=w214:dbl)
                n117 = for {
                  N: w208 -> [_]
                  tunnel: w214 -> [w220]
                  shift-right: [w215] -> w210
                  shift-left: _ -> [w218]
                  tunnel: w212 -> [w219]
                  i -> [w221]
                  n118 = Multiply(x=w220, y=w221) -> (x*y=w217:dbl)
                  n119 = Add(x=w219, y=w217) -> (x+y=w216:dbl)
                  n120 = Build Array (concatenate)(w218, w216) -> (w215:dbl[])
                }
              }
            }
            n121 = Build Array (concatenate)(w166, w174) -> (w165:dbl[][])
            n122 = call-poly <vilib>:"Plot Helper.vi"("z matrix"=w165, "y vector"=w162, "x vector"=w167) -> ("3D Plot lvclass Array out"=→"3D Surface":refnum<class "3D Plot Datatype.lvclass">[])  [unwired: 3 in, 5 out]
          }
        }
        frame #3 {
          n123 = property on="ramping step" class="DigNum (strict)"() -> ("Value"=w334:i32)  [unwired: 2 in, 2 out]
          n124 = Subtract(x=0.0, y=w337) -> (x-y=w344:dbl)
          n125 = Subtract(x=0.0, y=w335) -> (x-y=w342:dbl)
          n126 = property on="gate1 address" class="VISAName"() -> ("Value"=w345:refnum<visa-resource-name>)  [unwired: 2 in, 2 out]
          n127 = Divide(x=w344, y=w334) -> (x/y=w343:dbl)
          n128 = property on="Function (0: Volts) 2" class="Ring (strict)"() -> ("Value"=w339:u16)  [unwired: 2 in, 2 out]
          n129 = Divide(x=w342, y=w334) -> (x/y=w340:dbl)
          n130 = property on="gate2 address" class="VISAName"() -> ("Value"=w341:refnum<visa-resource-name>)  [unwired: 2 in, 2 out]
          n131 = Increment(x=w334) -> (x+1=w333:i32)
          n132 = for {
            N: w333 -> [_]
            tunnel: w339 -> [w355]
            tunnel: w345 -> [w354]
            tunnel: w337 -> [w353]
            tunnel: w343 -> [w352]
            tunnel: w341 -> [w349]
            tunnel: w335 -> [w346]
            tunnel: w340 -> [w347]
            tunnel: w339 -> [w350]
            i -> [w351]
            n133 = flat-sequence {
              tunnel: w355 -> [w374]
              tunnel: w354 -> [w372]
              tunnel: w353 -> [w371]
              tunnel: w352 -> [w370]
              tunnel: w351 -> [w368]
              tunnel: [w368] -> w348
              tunnel: w350 -> [w384]
              tunnel: w349 -> [w383]
              tunnel: w346 -> [w382]
              tunnel: [w380] -> _
              tunnel: w348 -> [w381]
              tunnel: w347 -> [w380]
              frame #0 {
                w356 = "defbuffer1" ("Buffer Name (defbuffer1) 2")
                w364 = "\""
                w361 = ":READ?"  # Read Measurement
                (unwired) u32 10000  # Bytes
                w378 = "VOLT\nCURR"  # Source Function
                w377 = ":SOUR:%s %g;"  # Manual Range
                # "SCPI 2450"
                n134 = Multiply(x=w368, y=w370) -> (x*y=w375:dbl)
                n135 = Wait (ms)(milliseconds to wait=50) -> ()  [unwired: 1 out]
                n136 = Add(x=w371, y=w375) -> (x+y=w373:dbl)
                n137 = Equal?(x="", y=w356) -> (x = y?=w358:bool)
                n138 = Select(t="defbuffer1", s=w358, f=w356) -> (s? t:f=w363:string)
                n139 = Pick Line(multi-line string=w378, line index=w374) -> (output string=w379:string)  [unwired: 1 out]
                n140 = call <vilib>:"Space Constant.vi"() -> ("String"=w362:string)
                n141 = Format Into String(format string=w377, w379, w373) -> (resulting string=w376:string)  [unwired: 2 in, 1 out]
                n142 = Concatenate Strings(w361, w362, w364, w363, w364, ", " ("string"), "READ" ("Buffer Elements 2")) -> (w367:string)
                n143 = VISA Write(VISA resource name=w372, write buffer=w376) -> (VISA resource name out=w357:refnum<visa-resource-name>)  [unwired: 1 in, 2 out]
                n144 = VISA Write(VISA resource name=w357, write buffer=w367) -> ()  [unwired: 1 in, 3 out]
              }
              frame #1 {
                n145 = Wait (ms)(milliseconds to wait=50) -> ()  [unwired: 1 out]
                n146 = Multiply(x=w380, y=w381) -> (x*y=w385:dbl)
                n147 = Add(x=w382, y=w385) -> (x+y=w386:dbl)
                n148 = call <instrlib>:"Configure Output.vi"("Source Mode  (0: Voltage)"=w384, "Output Level (0)"=w386, "VISA resource name"=w383) -> ()  [unwired: 7 in, 2 out]
              }
            }
          }
        }
      }
    }
  }
  n149 = call <instrlib>:"Initialize.vi"("Serial Configuration"="Serial Configuration", "VISA resource name"="gate2 address") -> ("error out"=w13:errorcluster, "VISA resource name out"=w14:refnum<visa-resource-name>)  [unwired: 8 in]
  n150 = call <instrlib>:"Configure Measurement.vi"("error in (no error)"=w13, "Enable Auto Range (T:Enable)"=w4, "Function (0: Volts)"=w8, "VISA resource name"=w14) -> ("error out"=w12:errorcluster, "VISA resource name out"=w11:refnum<visa-resource-name>)  [unwired: 6 in]
  n151 = Concatenate Strings("path (folder + filename)", ".txt") -> (w16:string)
  n152 = call <instrlib>:"Configure Measurement.vi"("error in (no error)"=w12, "Enable Auto Range (T:Enable)"=w4, "Function (0: Volts)"=w7, "VISA resource name"=w11) -> ("error out"=w5:errorcluster, "VISA resource name out"=w6:refnum<visa-resource-name>)  [unwired: 6 in]
  n153 = String To Path(string=w16) -> (path=w15:path)
  n154 = call <instrlib>:"Configure Measurement.vi"("error in (no error)"=w5, "Enable Auto Range (T:Enable)"=w4, "Function (0: Volts)"=w3, "VISA resource name"=w6) -> ("error out"=w1:errorcluster, "VISA resource name out"=w2:refnum<visa-resource-name>)  [unwired: 6 in]
